vi "Splash Screen State.vi"   [LabVIEW 2014]
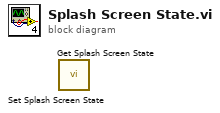
[diagram p0: block diagram]
diagram:
  n1 = call "Set Splash Screen State.vi"() -> ()  [unwired: 11 in, 1 out]
  n2 = call "Get Splash Screen State.vi"() -> ()  [unwired: 10 in, 2 out]
